vi "DataLogger.CheckAlarms.vi"(8 "error in (no error)":errorcluster, 9 "Value":string, 10 "DIM Service":string, 11 "i ref in":refnum<vi>) -> (0 "error out":errorcluster, 3 "i ref out":refnum<vi>)   [LabVIEW 2014, in "DataLogger.lvlib"]
uses:
  DataLogger.lvlib
  CSlibraries-extern/DimLVEvent/LVDimInterface/LVDimInterface.lvlib
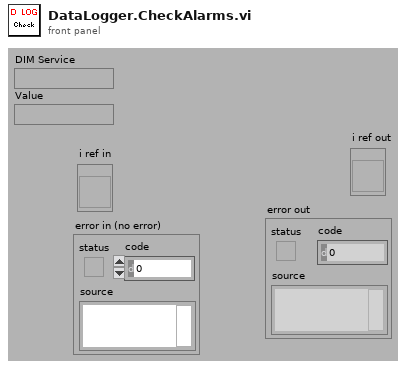
[diagram p1: front panel]
types:
  T1 = enum16{"open", "replace", "create", "open or create", "replace or create", "replace or create with confirmation"}
  T2 = typedef "DataLogger.lvlib/DataLogger.i attribute.ctl" = cluster{"Service Names":string[], "Path":string[], "Service Alarm Index":i32[], "Service Alarm Limit1":dbl[], "Service Alarm Limit2":dbl[], "Service Alarm Indicator":bool[], "alarmID":i32, "pathID":i32, "SoundDeviceID":i32, "SoundFile":string, "SoundID":i32, "SoundFileID":i32}
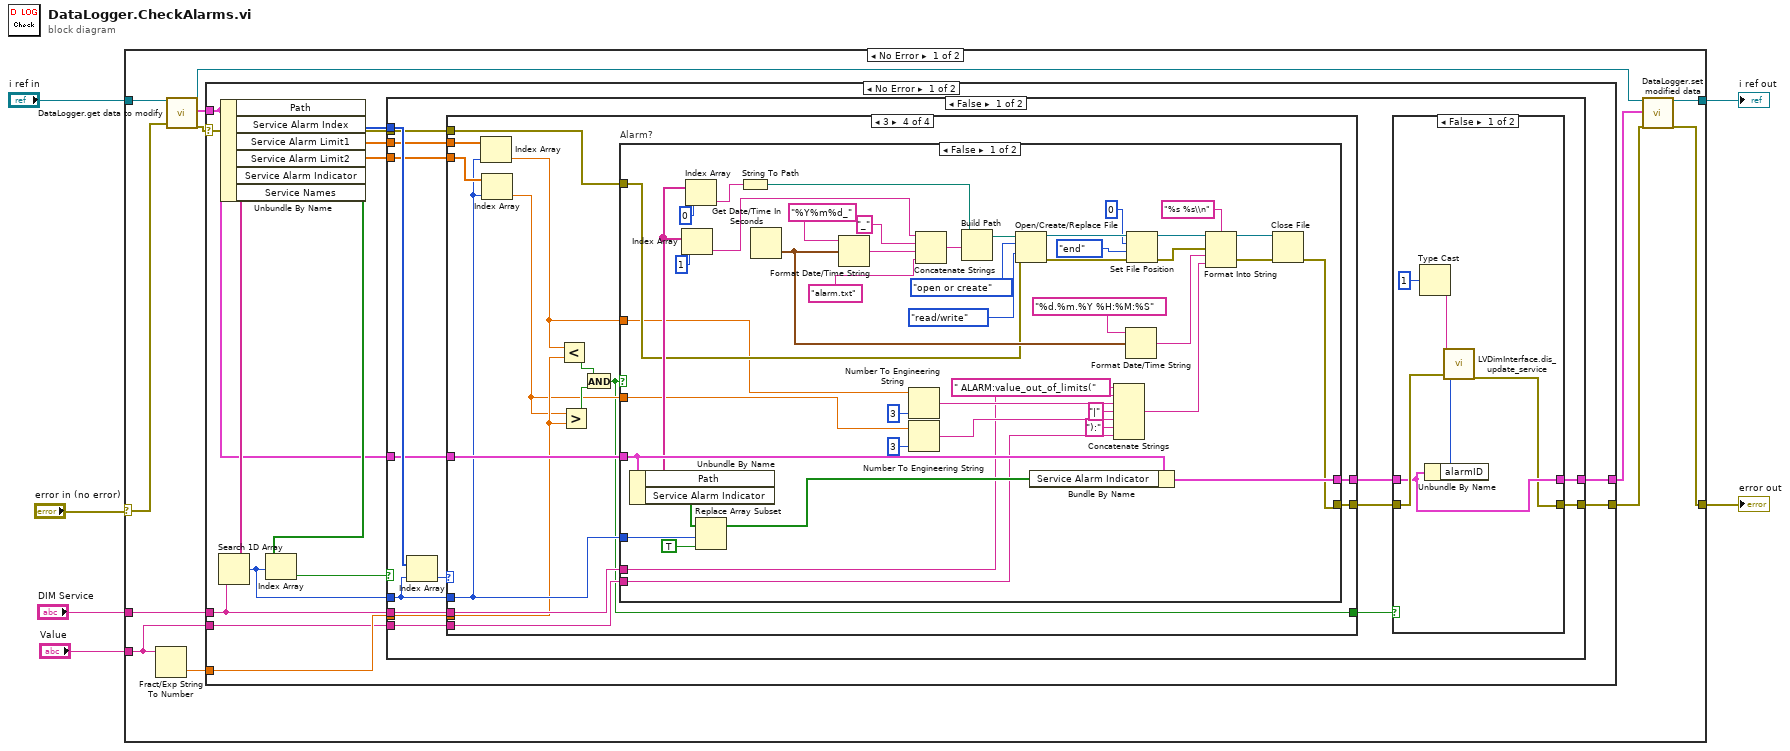
[diagram p0: block diagram]
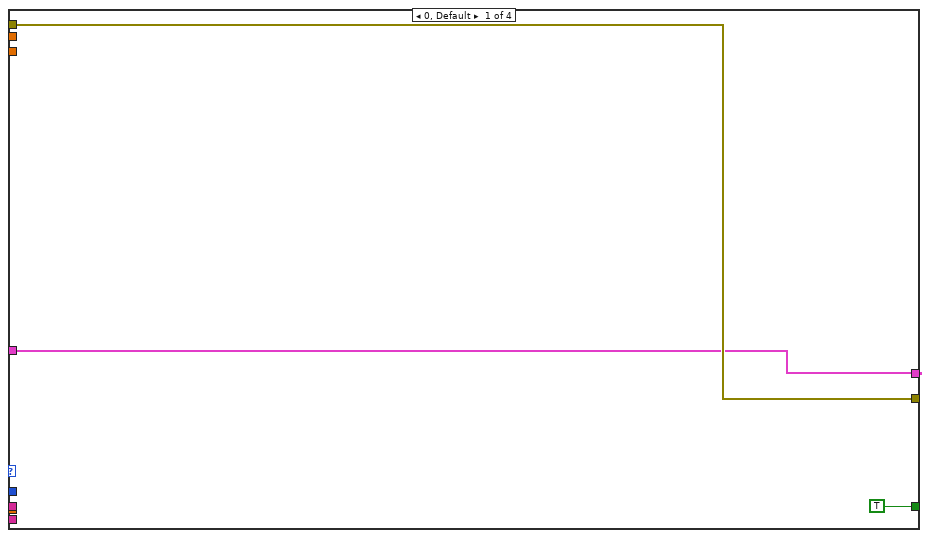
[diagram p3: hidden frame]
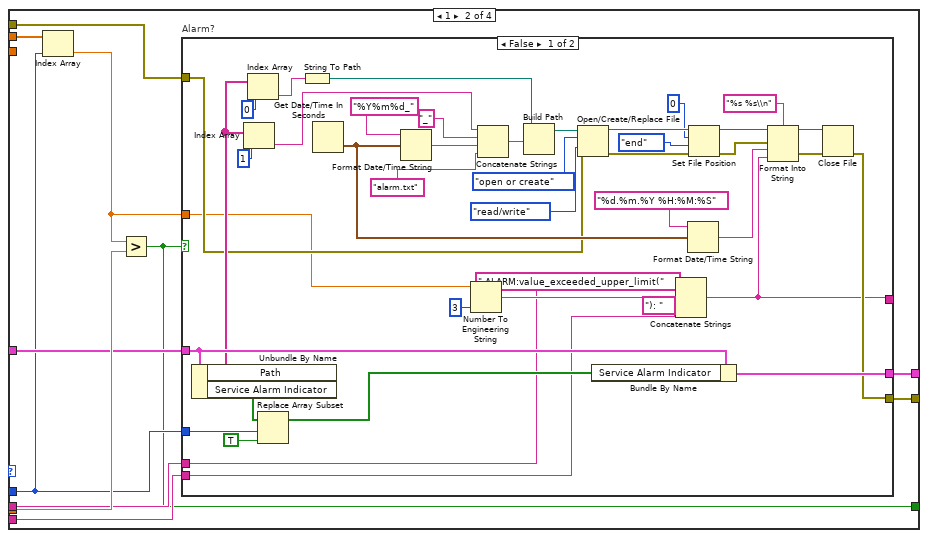
[diagram p4: hidden frame]
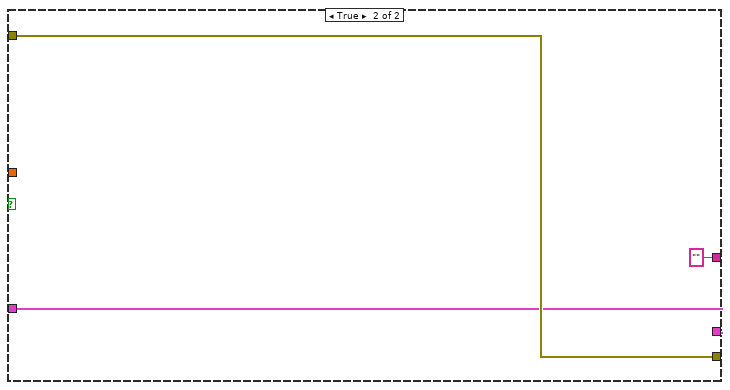
[diagram p5: hidden frame]
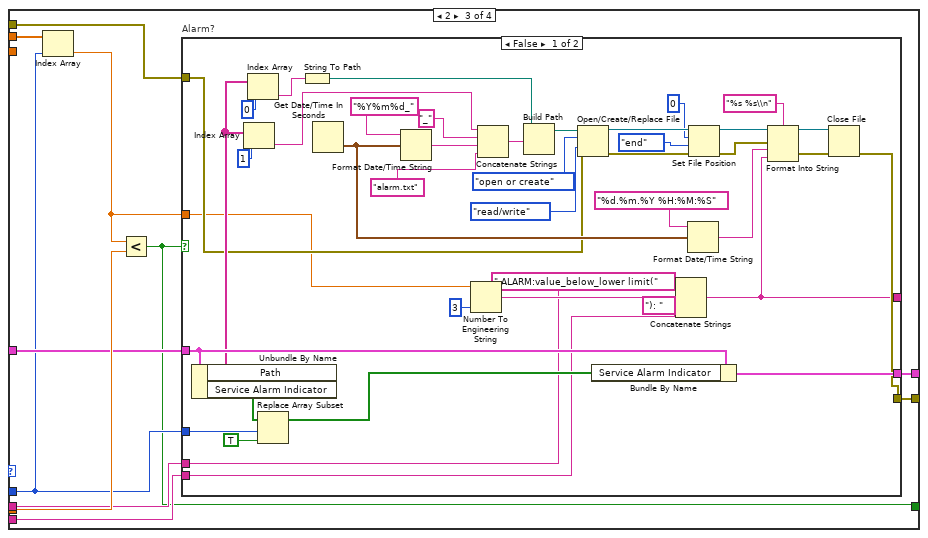
[diagram p6: hidden frame]
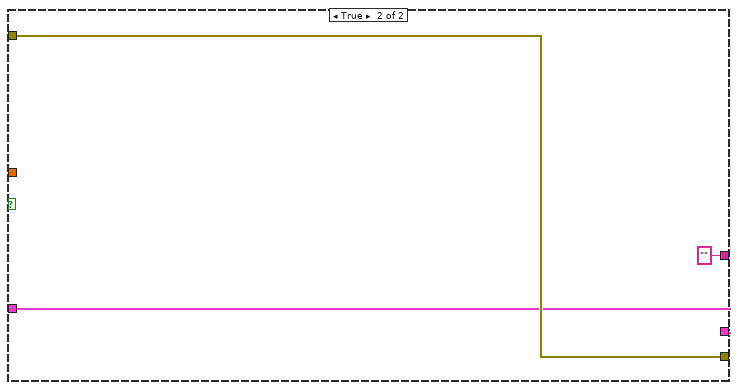
[diagram p7: hidden frame]
diagram:
  n1 = case shown="No Error" "error in (no error)" {
    selector: "error in (no error)" -> [w17 w238]
    tunnel: "i ref in" -> [w18 w239]
    tunnel: [w11 w239] -> w4
    tunnel: [w9 w238] -> w3
    tunnel: "DIM Service" -> [w15 _]
    tunnel: "Value" -> [w7 _]
    frame No Error {
      n2 = Fract/Exp String To Number(string=w7) -> (number=w13:dbl)  [unwired: 3 in, 1 out]
      n3 = call "DataLogger.get data to modify.vi"("i ref in"=w18, "error in (no error)"=w17) -> ("i ref out"=w12:refnum<vi>, "i attribute"=w16:T2, "error out"=w14:errorcluster)  [unwired: 14 in, 1 out]
      n4 = case shown="No Error" w14 {
        selector: w14 -> [w29 w237]
        tunnel: w16 -> [w23 w236]
        tunnel: w15 -> [w21 _]
        tunnel: [w28 w237] -> w10
        tunnel: w13 -> [w25 _]
        tunnel: [w22 w236] -> w8
        tunnel: w7 -> [w20 _]
        frame No Error {
          n5 = Unbundle By Name(w23) -> ("Service Alarm Index"=w26:i32[], "Service Alarm Limit1"=w24:dbl[], "Service Alarm Limit2"=w19:dbl[], "Service Alarm Indicator"=w31:bool[], "Service Names"=w32:string[])  [unwired: 1 out]
          n6 = Search 1D Array(1D array=w32, element=w21) -> (index of element=w27:i32)  [unwired: 1 in]
          n7 = Index Array(array=w31, index=w27) -> (element=w30:bool)
          n8 = case shown="False" w30 {
            tunnel: w29 -> [w45 w235]
            tunnel: [w33 w235] -> w28
            tunnel: w27 -> [w42 _]
            tunnel: w26 -> [w47 _]
            tunnel: w25 -> [w44 _]
            tunnel: w24 -> [w43 _]
            tunnel: w23 -> [w41 w234]
            tunnel: [w35 w234] -> w22
            tunnel: w21 -> [w40 _]
            tunnel: w20 -> [w39 _]
            tunnel: w19 -> [w38 _]
            frame False {
              n9 = Index Array(array=w47, index=w42) -> (element=w46:i32)
              n10 = case shown="3" w46 {
                tunnel: w45 -> [w58 w67 w123 w184]
                tunnel: [w58 w66 w122 w183] -> w34
                tunnel: w44 -> [_ w68 w124 w175]
                tunnel: w43 -> [_ w69 w125 w185]
                tunnel: w42 -> [_ w63 w119 w176]
                tunnel: w41 -> [w57 w65 w121 w182]
                tunnel: [w57 w64 w120 w181] -> w36
                tunnel: w40 -> [_ w62 w118 w180]
                tunnel: w39 -> [_ w60 w116 w178]
                tunnel: w38 -> [_ _ _ w177]
                tunnel: [TRUE w59 w115 w171] -> w37
                frame 0, Default {
                }
                frame 1 {
                  n11 = Index Array(array=w69, index=w63) -> (element=w61:dbl)
                  n12 = Greater?(x=w61, y=w68) -> (0:w59:bool)
                  n13 = case "Alarm?" shown="False" w59 {
                    tunnel: w67 -> [w81 w114]
                    tunnel: [w72 w114] -> w66
                    tunnel: w65 -> [w110 w113]
                    tunnel: [w111 w113] -> w64
                    tunnel: w63 -> [w108 _]
                    tunnel: w62 -> [w71 _]
                    tunnel: w61 -> [w78 _]
                    tunnel: w60 -> [w73 _]
                    tunnel: [w70 ""] -> _
                    frame False {
                      n14 = Unbundle By Name(w110) -> ("Path"=w102:string[], "Service Alarm Indicator"=w109:bool[])
                      n15 = Index Array(array=w102, index=1 ("length")) -> (element=w79:string)
                      n16 = Index Array(array=w102, index=0 ("length")) -> (element=w104:string)
                      n17 = Replace Array Subset(array=w109, new element=TRUE ("new element/subarray"), index=w108) -> (w106:bool[])
                      n18 = String To Path(string=w104) -> (path=w80:path)
                      n19 = Get Date/Time In Seconds() -> (seconds since 1Jan1904=w85:timestamp)
                      n20 = Format Date/Time String(time format string (%c)="%Y%m%d_", seconds (now)=w85) -> (date/time string=w99:string)  [unwired: 1 in]
                      n21 = Number To Engineering String(2:i16 3 ("precision (6)"), 4:w78) -> (0:w76:string)  [unwired: 2 in]
                      n22 = Concatenate Strings(w79, "_" ("string"), w99, "alarm.txt" ("string")) -> (w101:string)
                      n23 = Build Path(base path=w80, name or relative path=w101) -> (appended path=w92:path)
                      n24 = Open/Create/Replace File(file path (use dialog)=w92, error in=w81, operation (0:open)=T1."open or create", access (0:read/write)=enum16{"read/write", "read-only", "write-only"}."read/write") -> (refnum out=w91:refnum<file>, error out=w90:errorcluster)  [unwired: 2 in, 1 out]
                      n25 = Bundle By Name(cluster=w110, "Service Alarm Indicator"=w106) -> (w111:T2)
                      n26 = Concatenate Strings(w71, " ALARM:value_exceeded_upper_limit(" ("string"), w76, "): " ("string"), w73) -> (w70:string)
                      n27 = Format Date/Time String(time format string (%c)="%d.%m.%Y %H:%M:%S", seconds (now)=w85) -> (date/time string=w83:string)  [unwired: 1 in]
                      n28 = Set File Position(offset (in bytes) (0)=i64 0, refnum=w91, from (0:start)=enum16{"start", "end", "current"}."end", error in=w90) -> (refnum out=w88:refnum<file>, error out=w89:errorcluster)
                      n29 = Format Into String(format string="%s %s\\n", initial string=w88, error in=w89, w83, w70) -> (resulting string=w95:refnum<file>, error out=w96:errorcluster)
                      n30 = Close File(refnum=w95, error in=w96) -> (error out=w72:errorcluster)  [unwired: 1 out]
                    }
                    frame True {
                    }
                  }
                }
                frame 2 {
                  n31 = Index Array(array=w125, index=w119) -> (element=w117:dbl)
                  n32 = Less?(x=w117, y=w124) -> (x < y?=w115:bool)
                  n33 = case "Alarm?" shown="False" w115 {
                    tunnel: w123 -> [w137 w170]
                    tunnel: [w128 w170] -> w122
                    tunnel: w121 -> [w166 w169]
                    tunnel: [w167 w169] -> w120
                    tunnel: w119 -> [w164 _]
                    tunnel: w118 -> [w127 _]
                    tunnel: w117 -> [w134 _]
                    tunnel: w116 -> [w129 _]
                    tunnel: [w126 ""] -> _
                    frame False {
                      n34 = Unbundle By Name(w166) -> ("Path"=w158:string[], "Service Alarm Indicator"=w165:bool[])
                      n35 = Index Array(array=w158, index=1 ("length")) -> (element=w135:string)
                      n36 = Index Array(array=w158, index=0 ("length")) -> (element=w160:string)
                      n37 = Replace Array Subset(array=w165, new element=TRUE ("new element/subarray"), index=w164) -> (w162:bool[])
                      n38 = String To Path(string=w160) -> (path=w136:path)
                      n39 = Get Date/Time In Seconds() -> (seconds since 1Jan1904=w141:timestamp)
                      n40 = Format Date/Time String(time format string (%c)="%Y%m%d_", seconds (now)=w141) -> (date/time string=w155:string)  [unwired: 1 in]
                      n41 = Number To Engineering String(2:i16 3 ("precision (6)"), 4:w134) -> (0:w132:string)  [unwired: 2 in]
                      n42 = Concatenate Strings(w135, "_" ("string"), w155, "alarm.txt" ("string")) -> (w157:string)
                      n43 = Build Path(base path=w136, name or relative path=w157) -> (appended path=w148:path)
                      n44 = Open/Create/Replace File(file path (use dialog)=w148, error in=w137, operation (0:open)=T1."open or create", access (0:read/write)=enum16{"read/write", "read-only", "write-only"}."read/write") -> (refnum out=w147:refnum<file>, error out=w146:errorcluster)  [unwired: 2 in, 1 out]
                      n45 = Bundle By Name(cluster=w166, "Service Alarm Indicator"=w162) -> (w167:T2)
                      n46 = Concatenate Strings(w127, " ALARM:value_below_lower limit(" ("string"), w132, "): " ("string"), w129) -> (w126:string)
                      n47 = Format Date/Time String(time format string (%c)="%d.%m.%Y %H:%M:%S", seconds (now)=w141) -> (date/time string=w139:string)  [unwired: 1 in]
                      n48 = Set File Position(offset (in bytes) (0)=i64 0, refnum=w147, from (0:start)=enum16{"start", "end", "current"}."end", error in=w146) -> (refnum out=w144:refnum<file>, error out=w145:errorcluster)
                      n49 = Format Into String(format string="%s %s\\n", initial string=w144, error in=w145, w139, w126) -> (resulting string=w151:refnum<file>, error out=w152:errorcluster)
                      n50 = Close File(refnum=w151, error in=w152) -> (error out=w128:errorcluster)  [unwired: 1 out]
                    }
                    frame True {
                    }
                  }
                }
                frame 3 {
                  n51 = Index Array(array=w185, index=w176) -> (element=w179:dbl)
                  n52 = Index Array(array=w177, index=w176) -> (element=w172:dbl)
                  n53 = Less?(x=w179, y=w175) -> (x < y?=w174:bool)
                  n54 = Greater?(x=w172, y=w175) -> (0:w173:bool)
                  n55 = And(x=w174, y=w173) -> (x .and. y?=w171:bool)
                  n56 = case "Alarm?" shown="False" w171 {
                    tunnel: w184 -> [w202 w233]
                    tunnel: [w195 w233] -> w183
                    tunnel: w182 -> [w230 w232]
                    tunnel: [w231 w232] -> w181
                    tunnel: w176 -> [w228 _]
                    tunnel: w180 -> [w187 _]
                    tunnel: w179 -> [w199 _]
                    tunnel: w178 -> [w192 _]
                    tunnel: w172 -> [w193 _]
                    frame False {
                      n57 = Unbundle By Name(w230) -> ("Path"=w222:string[], "Service Alarm Indicator"=w229:bool[])
                      n58 = Index Array(array=w222, index=1 ("length")) -> (element=w200:string)
                      n59 = Index Array(array=w222, index=0 ("length")) -> (element=w224:string)
                      n60 = Replace Array Subset(array=w229, new element=TRUE ("new element/subarray"), index=w228) -> (w226:bool[])
                      n61 = String To Path(string=w224) -> (path=w201:path)
                      n62 = Get Date/Time In Seconds() -> (seconds since 1Jan1904=w206:timestamp)
                      n63 = Format Date/Time String(time format string (%c)="%Y%m%d_", seconds (now)=w206) -> (date/time string=w219:string)  [unwired: 1 in]
                      n64 = Number To Engineering String(2:i16 3 ("precision (6)"), 4:w199) -> (0:w197:string)  [unwired: 2 in]
                      n65 = Number To Engineering String(2:i16 3 ("precision (6)"), 4:w193) -> (0:w190:string)  [unwired: 2 in]
                      n66 = Concatenate Strings(w200, "_" ("string"), w219, "alarm.txt" ("string")) -> (w221:string)
                      n67 = Build Path(base path=w201, name or relative path=w221) -> (appended path=w213:path)
                      n68 = Open/Create/Replace File(file path (use dialog)=w213, error in=w202, operation (0:open)=T1."open or create", access (0:read/write)=enum16{"read/write", "read-only", "write-only"}."read/write") -> (refnum out=w212:refnum<file>, error out=w211:errorcluster)  [unwired: 2 in, 1 out]
                      n69 = Bundle By Name(cluster=w230, "Service Alarm Indicator"=w226) -> (w231:T2)
                      n70 = Concatenate Strings(w187, " ALARM:value_out_of_limits(" ("string"), w197, "|" ("string"), w190, "):" ("string"), w192) -> (w186:string)
                      n71 = Format Date/Time String(time format string (%c)="%d.%m.%Y %H:%M:%S", seconds (now)=w206) -> (date/time string=w204:string)  [unwired: 1 in]
                      n72 = Set File Position(offset (in bytes) (0)=i64 0, refnum=w212, from (0:start)=enum16{"start", "end", "current"}."end", error in=w211) -> (refnum out=w209:refnum<file>, error out=w210:errorcluster)
                      n73 = Format Into String(format string="%s %s\\n", initial string=w209, error in=w210, w204, w186) -> (resulting string=w216:refnum<file>, error out=w188:errorcluster)
                      n74 = Close File(refnum=w216, error in=w188) -> (error out=w195:errorcluster)  [unwired: 1 out]
                    }
                    frame True {
                    }
                  }
                }
              }
              n75 = case shown="False" w37 {
                tunnel: w36 -> [w52 w55]
                tunnel: [w52 w55] -> w35
                tunnel: w34 -> [w53 w54]
                tunnel: [w48 w54] -> w33
                frame False {
                  n76 = Type Cast(x=1) -> (*(type *) &x=w49:string)  [unwired: 1 in]
                  n77 = Unbundle By Name(w52) -> ("alarmID"=w51:i32)
                  n78 = call "LVDimInterface.dis_update_service.vi"("my_serviceID"=w51, "data"=w49, "error in (no error)"=w53) -> ("error out"=w48:errorcluster)  [unwired: 14 in, 2 out]
                }
                frame True {
                }
              }
            }
            frame True {
            }
          }
        }
        frame Error {
        }
      }
      n79 = call "DataLogger.set modified data.vi"("i ref in"=w12, "i attribute"=w8, "error in (no error)"=w10) -> ("i ref out"=w11:refnum<vi>, "error out"=w9:errorcluster)  [unwired: 15 in]
    }
    frame Error {
    }
  }
  "error out" <- w3
  "i ref out" <- w4
